vi "Create Steering Frame.vi"   [LabVIEW 2017, in "NI_Robotics_Steering Frame.lvclass"]
doc: "Creates a steering frame of the type you specify. You must manually select the polymorphic instance to use."
uses:
  <vilib>/robotics/Steering/Steering Frame/NI_Robotics_Steering Frame.lvclass
  <vilib>/robotics/Steering/Differential Steering Frame/NI_Robotics_Differential Steering Frame.lvclass
  <vilib>/robotics/Steering/Ackermann Steering Frame/NI_Robotics_Ackermann Steering Frame.lvclass
  <vilib>/robotics/Steering/Mecanum Steering Frame/NI_Robotics_Mecanum Steering Frame.lvclass
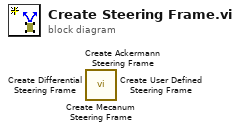
[diagram p0: block diagram]
diagram:
  n1 = call <vilib>:"Create Mecanum Steering Frame.vi"() -> ()  [unwired: 10 in, 2 out]
  n2 = call <vilib>:"Create Ackermann Steering Frame.vi"() -> ()  [unwired: 10 in, 2 out]
  n3 = call <vilib>:"Create Differential Steering Frame.vi"() -> ()  [unwired: 10 in, 2 out]
  n4 = call <vilib>:"Create User Defined Steering Frame.vi"() -> ()  [unwired: 10 in, 2 out]
